vi "sub_DWA_calc-control-n-trajectory.vi"(11 "dw":dbl[](array[numeric])) -> (2 "best trajectory":dbl[][](array[numeric]), 3 "u":cluster{"v":dbl, "y":dbl} {"y" format="%.18f"; "v" format="%.19f"})   [LabVIEW 2019]
uses:
  Ctrl/cmd_common.ctl
panel:
  out "vn loop":i32
  out "yn loop":i32
  out "yn":dbl
  out "vn":dbl
  out "x_init":dbl[](array[numeric])
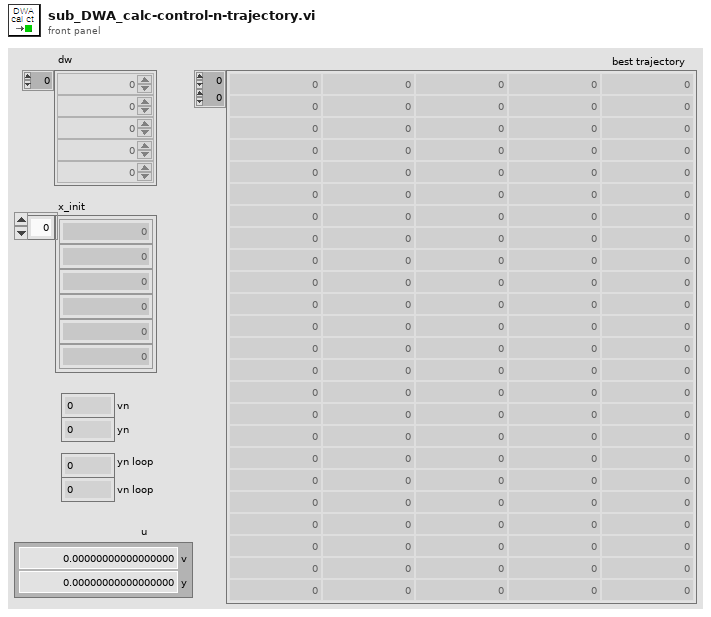
[diagram p1: front panel]
types:
  T1 = typedef "cmd_common.ctl" = enum16{"read", "write"}
  T2 = cluster{"x":dbl[], "dw":dbl[], "u":cluster{"v":dbl, "y":dbl}, "trajectory":dbl[][], "best trajectory":dbl[][], "best u":cluster{"v":dbl, "y":dbl}, "cost":cluster{"goal":dbl, "speed":dbl, "obstacle":dbl, "final":dbl}}
  T3 = cluster{"max speed":dbl, "min speed":dbl, "max yaw rate":dbl, "max accel":dbl, "max delta yaw rate":dbl, "v resolution":dbl, "yaw rate resolution":dbl, "dt":dbl, "predict time":dbl, "to goal cost gain":dbl, "speed cost gain":dbl, "obstacle cost gain":dbl, "robot stuck flag cons":dbl, "robot type":enum16{"circle", "rectangle"}, "robot radius":dbl, "robot width":dbl, "robot length":dbl, "obstacles":cluster{"x":dbl, "y":dbl}[], "goal pt":cluster{"x":i32, "y":i32}}
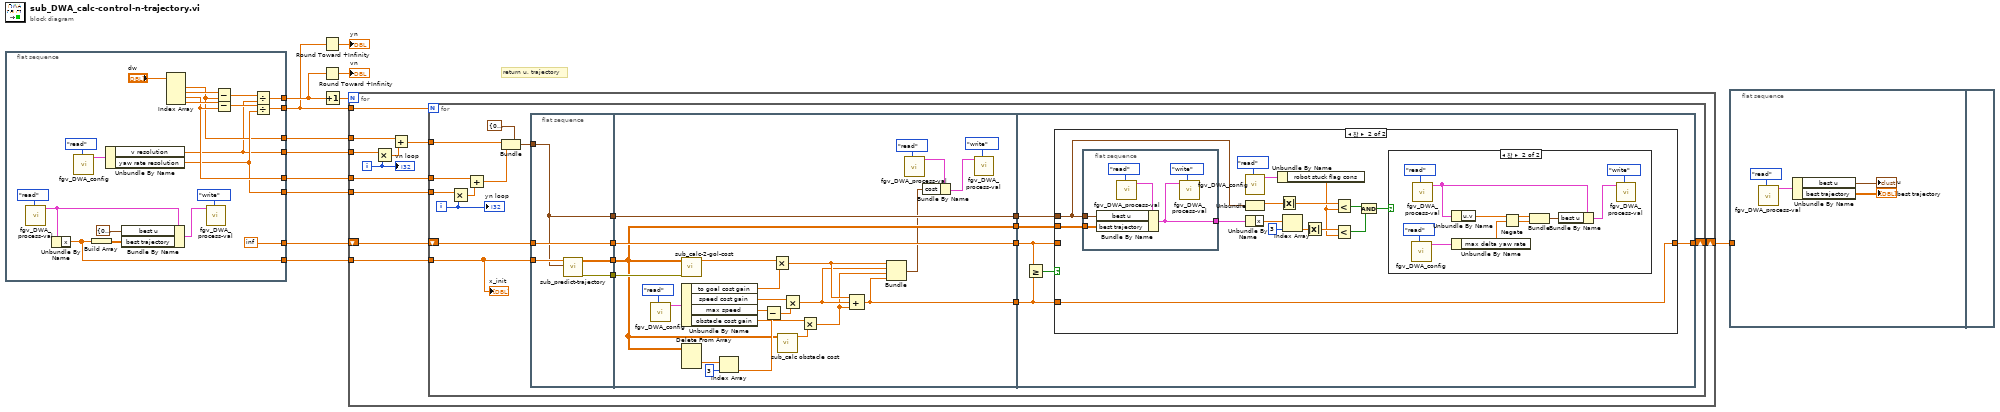
[diagram p0: block diagram]
diagram:
  # "return u, trajectory"
  n1 = flat-sequence {
    tunnel: [w29] -> w4
    tunnel: [w26] -> w1
    tunnel: [w25] -> w12
    tunnel: [w24] -> w11
    tunnel: [inf] -> w10
    tunnel: [w22] -> w9
    tunnel: [w21] -> w8
    tunnel: [w13] -> w7
    frame #0 {
      n2 = call "fgv_DWA_process-val.vi"("cmd"=cmd_common."read") -> ("prcess val out"=w16:T2)  [unwired: 10 in]
      n3 = Unbundle By Name(w16) -> ("x"=w13:dbl[])
      n4 = call "fgv_DWA_config.vi"("cmd"=cmd_common."read") -> ("config out"=w32:T3)  [unwired: 10 in]
      n5 = Build Array(w13) -> (w15:dbl[][])
      n6 = Unbundle By Name(w32) -> ("v resolution"=w21:dbl, "yaw rate resolution"=w24:dbl)
      n7 = Bundle By Name(cluster=w16, "best u"=cluster{"v":dbl, "y":dbl} {"v"=0.0, "y"=0.0}, "best trajectory"=w15) -> (w17:T2)
      n8 = Index Array(array="dw") -> (element #1=w22:dbl, element #2=w31:dbl, element #3=w25:dbl, element #4=w27:dbl)  [unwired: 4 in]
      n9 = call "fgv_DWA_process-val.vi"("cmd"=cmd_common."write", "prcess val"=w17) -> ()  [unwired: 9 in, 1 out]
      n10 = Subtract(x=w31, y=w22) -> (x-y=w30:dbl)
      n11 = Subtract(x=w27, y=w25) -> (x-y=w28:dbl)
      n12 = Divide(x=w30, y=w21) -> (x/y=w29:dbl)
      n13 = Divide(x=w28, y=w24) -> (x/y=w26:dbl)
    }
  }
  n14 = Round Toward +Infinity(x=w1) -> (ceil(x): smallest int >= x=→"yn":dbl)
  n15 = Round Toward +Infinity(x=w4) -> (ceil(x): smallest int >= x=→"vn":dbl)
  n16 = Increment(x=w4) -> (x+1=w5:dbl)
  n17 = for {
    N: w5 -> [_]
    tunnel: w1 -> [w44]
    tunnel: w12 -> [w43]
    tunnel: w11 -> [w42]
    shift-right: [w40] -> w6
    shift-left: w10 -> [w41]
    tunnel: w9 -> [w34]
    tunnel: w8 -> [w35]
    tunnel: w7 -> [w39]
    i -> [w36]
    n18 = Multiply(x=w35, y=w36) -> (x*y=w38:dbl)
    n19 = Add(x=w34, y=w38) -> (x+y=w37:dbl)
    n20 = for {
      N: w44 -> [_]
      tunnel: w43 -> [w63]
      tunnel: w42 -> [w61]
      shift-right: [w51] -> w40
      shift-left: w41 -> [w54]
      tunnel: w39 -> [w46]
      tunnel: w37 -> [w45]
      i -> [w62]
      n21 = Multiply(x=w61, y=w62) -> (x*y=w60:dbl)
      n22 = Add(x=w63, y=w60) -> (x+y=w59:dbl)
      n23 = Bundle(cluster=cluster{"v":dbl, "u":dbl} {"v"=0.0, "u"=0.0} ("vy"), "v"=w45, "u"=w59) -> (w56:cluster{"v":dbl, "u":dbl})
      n24 = flat-sequence {
        tunnel: [w67] -> w57
        tunnel: w56 -> [w65]
        tunnel: w46 -> [w68]
        tunnel: w54 -> [w66]
        tunnel: [w66] -> w53
        tunnel: [w65] -> w49
        tunnel: [w64] -> w47
        tunnel: w57 -> [w93]
        tunnel: [w70] -> w55
        tunnel: w53 -> [w80]
        tunnel: [w80] -> w52
        tunnel: [w79] -> w50
        tunnel: w49 -> [w79]
        tunnel: [w78] -> w48
        tunnel: w47 -> [w78]
        tunnel: w55 -> [w97]
        tunnel: w52 -> [w96]
        tunnel: [w98] -> w51
        tunnel: w50 -> [w95]
        tunnel: w48 -> [w94]
        frame #0 {
          n25 = call "sub_predict-trajectory.vi"("u"=w65, "x"=w68) -> ("error out"=w67:errorcluster, "trajectory"=w64:dbl[][])  [unwired: 8 in]
        }
        frame #1 {
          n26 = call "fgv_DWA_config.vi"("cmd"=cmd_common."read") -> ("config out"=w91:T3)  [unwired: 10 in]
          n27 = call "sub_calc-2-gol-cost.vi"("error in"=w93, "trajectory"=w78) -> ("cost"=w89:dbl)  [unwired: 8 in, 1 out]
          n28 = Unbundle By Name(w91) -> ("to goal cost gain"=w90:dbl, "speed cost gain"=w88:dbl, "max speed"=w87:dbl, "obstacle cost gain"=w82:dbl)
          n29 = Delete From Array(array=w78) -> (deleted portion=w86:dbl[])  [unwired: 3 in, 1 out]
          n30 = Index Array(array=w86, index=3) -> (element=w84:dbl)
          n31 = Subtract(x=w87, y=w84) -> (x-y=w83:dbl)
          n32 = Multiply(x=w89, y=w90) -> (x*y=w73:dbl)
          n33 = call "sub_calc obstacle cost.vi"("trajectory"=w78) -> ("cost"=w81:dbl)  [unwired: 10 in]
          n34 = Multiply(x=w88, y=w83) -> (x*y=w72:dbl)
          n35 = Multiply(x=w82, y=w81) -> (x*y=w71:dbl)
          n36 = Compound Arithmetic op=ADD(w73, w72, w71) -> (w70:dbl)
          n37 = Bundle(w73, w72, w71, w70) -> (w69:cluster{dbl, dbl, dbl, dbl})  [unwired: 1 in]
          n38 = call "fgv_DWA_process-val.vi"("cmd"=cmd_common."read") -> ("prcess val out"=w76:T2)  [unwired: 10 in]
          n39 = Bundle By Name(cluster=w76, "cost"=w69) -> (w77:T2)
          n40 = call "fgv_DWA_process-val.vi"("cmd"=cmd_common."write", "prcess val"=w77) -> ()  [unwired: 9 in, 1 out]
        }
        frame #2 {
          n41 = Greater Or Equal?(x=w96, y=w97) -> (x >= y?=w99:bool)
          n42 = case shown="참" w99 {
            tunnel: [w100 w116] -> w98
            tunnel: w97 -> [_ w116]
            tunnel: w96 -> [w100 _]
            tunnel: w95 -> [_ w111]
            tunnel: w94 -> [_ w115]
            frame False {
            }
            frame True {
              n43 = flat-sequence {
                tunnel: w111 -> [w129]
                tunnel: w115 -> [w128]
                tunnel: [w127] -> w110
                frame #0 {
                  n44 = call "fgv_DWA_process-val.vi"("cmd"=cmd_common."read") -> ("prcess val out"=w132:T2)  [unwired: 10 in]
                  n45 = Bundle By Name(cluster=w132, "best u"=w129, "best trajectory"=w128) -> (w127:T2)
                  n46 = call "fgv_DWA_process-val.vi"("cmd"=cmd_common."write", "prcess val"=w127) -> ()  [unwired: 9 in, 1 out]
                }
              }
              n47 = call "fgv_DWA_config.vi"("cmd"=cmd_common."read") -> ("config out"=w112:T3)  [unwired: 10 in]
              n48 = Unbundle(w111) -> ("v"=w114:dbl)  [unwired: 1 out]
              n49 = Unbundle By Name(w110) -> ("x"=w109:dbl[])
              n50 = Unbundle By Name(w112) -> ("robot stuck flag cons"=w101:dbl)
              n51 = Absolute Value(x=w114) -> (abs(x)=w102:dbl)
              n52 = Index Array(array=w109, index=3 ("인덱스")) -> (element=w107:dbl)
              n53 = Absolute Value(x=w107) -> (abs(x)=w103:dbl)
              n54 = Less?(x=w102, y=w101) -> (x < y?=w106:bool)
              n55 = Less?(x=w103, y=w101) -> (x < y?=w105:bool)
              n56 = And(x=w106, y=w105) -> (x .and. y?=w104:bool)
              n57 = case shown="참" w104 {
                frame False {
                }
                frame True {
                  n58 = call "fgv_DWA_config.vi"("cmd"=cmd_common."read") -> ("config out"=w123:T3)  [unwired: 10 in]
                  n59 = call "fgv_DWA_process-val.vi"("cmd"=cmd_common."read") -> ("prcess val out"=w121:T2)  [unwired: 10 in]
                  n60 = Unbundle By Name(w121) -> ("u.v"=w119:dbl)
                  n61 = Unbundle By Name(w123) -> ("max delta yaw rate"=w118:dbl)
                  n62 = Negate(x=w118) -> (-x=w117:dbl)
                  n63 = Bundle("v"=w119, w117) -> (w120:cluster{"v":dbl, dbl})  [unwired: 1 in]
                  n64 = Bundle By Name(cluster=w121, "best u"=w120) -> (w126:T2)
                  n65 = call "fgv_DWA_process-val.vi"("cmd"=cmd_common."write", "prcess val"=w126) -> ()  [unwired: 9 in, 1 out]
                }
              }
            }
          }
        }
      }
      "x_init" <- w46
      "yn loop" <- w62
    }
    "vn loop" <- w36
  }
  n66 = flat-sequence {
    tunnel: w6 -> [_]
    frame #0 {
      n67 = call "fgv_DWA_process-val.vi"("cmd"=cmd_common."read") -> ("prcess val out"=w135:T2)  [unwired: 10 in]
      n68 = Unbundle By Name(w135) -> ("best u"=→"u":cluster{"v":dbl, "y":dbl}, "best trajectory"=→"best trajectory":dbl[][])
    }
    frame #1 {
    }
  }
